vi "Log BoP.vi"(9 "Stop Chat":bool, 10 "Send":bool, 11 "Enter Text":string) -> (3 "Chat Window":string)   [LabVIEW 2017]
uses:
  <vilib>/OPCUA/controls/Write Status.ctl
  <vilib>/OPCUA/controls/NodeId.ctl
  <vilib>/OPCUA/client/Multiple Write String.vi
  <vilib>/OPCUA/NI OPC UA Client.lvlib
panel:
  out "Log Loop":i32
  out "Send Loop":i32
  in  "Node Status":T1 items=["Good"=0, "Uncertain_InitialValue"=1083310080, "Uncertain_LastUsableValue"=1083179008, "Uncertain_SensorNotAccurate"=1083375616, "Uncertain_EngineeringUnitsExceeded"=1083441152, "Bad_NoCommunication"=2150694912, "Bad_NotReadable"=2151284736, "Bad_NotWritable"=2151350272, "Bad_OutOfRange"=2151415808, "Bad_WaitingForInitialData"=2150760448]
  in  "Time Stamp":timestamp
  in  "Node Status":T1 items=["Good"=0, "Uncertain_InitialValue"=1083310080, "Uncertain_LastUsableValue"=1083179008, "Uncertain_SensorNotAccurate"=1083375616, "Uncertain_EngineeringUnitsExceeded"=1083441152, "Bad_NoCommunication"=2150694912, "Bad_NotReadable"=2151284736, "Bad_NotWritable"=2151350272, "Bad_OutOfRange"=2151415808, "Bad_WaitingForInitialData"=2150760448]
  in  "Time Stamp":timestamp
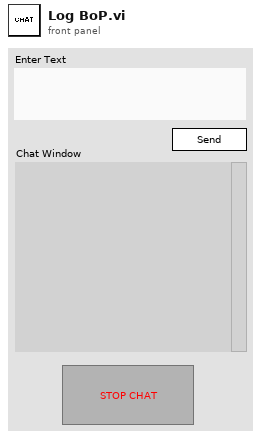
[diagram p1: front panel]
types:
  T1 = typedef "Write Status.ctl" = u32
  T2 = enum16{"open", "replace", "create", "open or create", "replace or create", "replace or create with confirmation"}
  T3 = typedef "OPC UA Client Refnum.ctl" = refnum<k21>
  T4 = typedef "NodeId.ctl" = string
  T5 = cluster{"node ID":T4, "value":string, "timestamp (current time)":timestamp, "node status":T1}
  T6 = cluster{"node ID":T4, "value":string, "timestamp (current time)":timestamp, "node status":T1}[]
  T7 = typedef "Subscription ID.ctl" = u32
  T8 = typedef "Subscription Data Change.ctl" = cluster{"node ID":T4, " value":variant, "timestamp":timestamp, "data type":T9, "status code":T10}
  T9 = typedef "Data Type.ctl" = u16
  T10 = typedef "OPC UA StatusCode.ctl" = u32
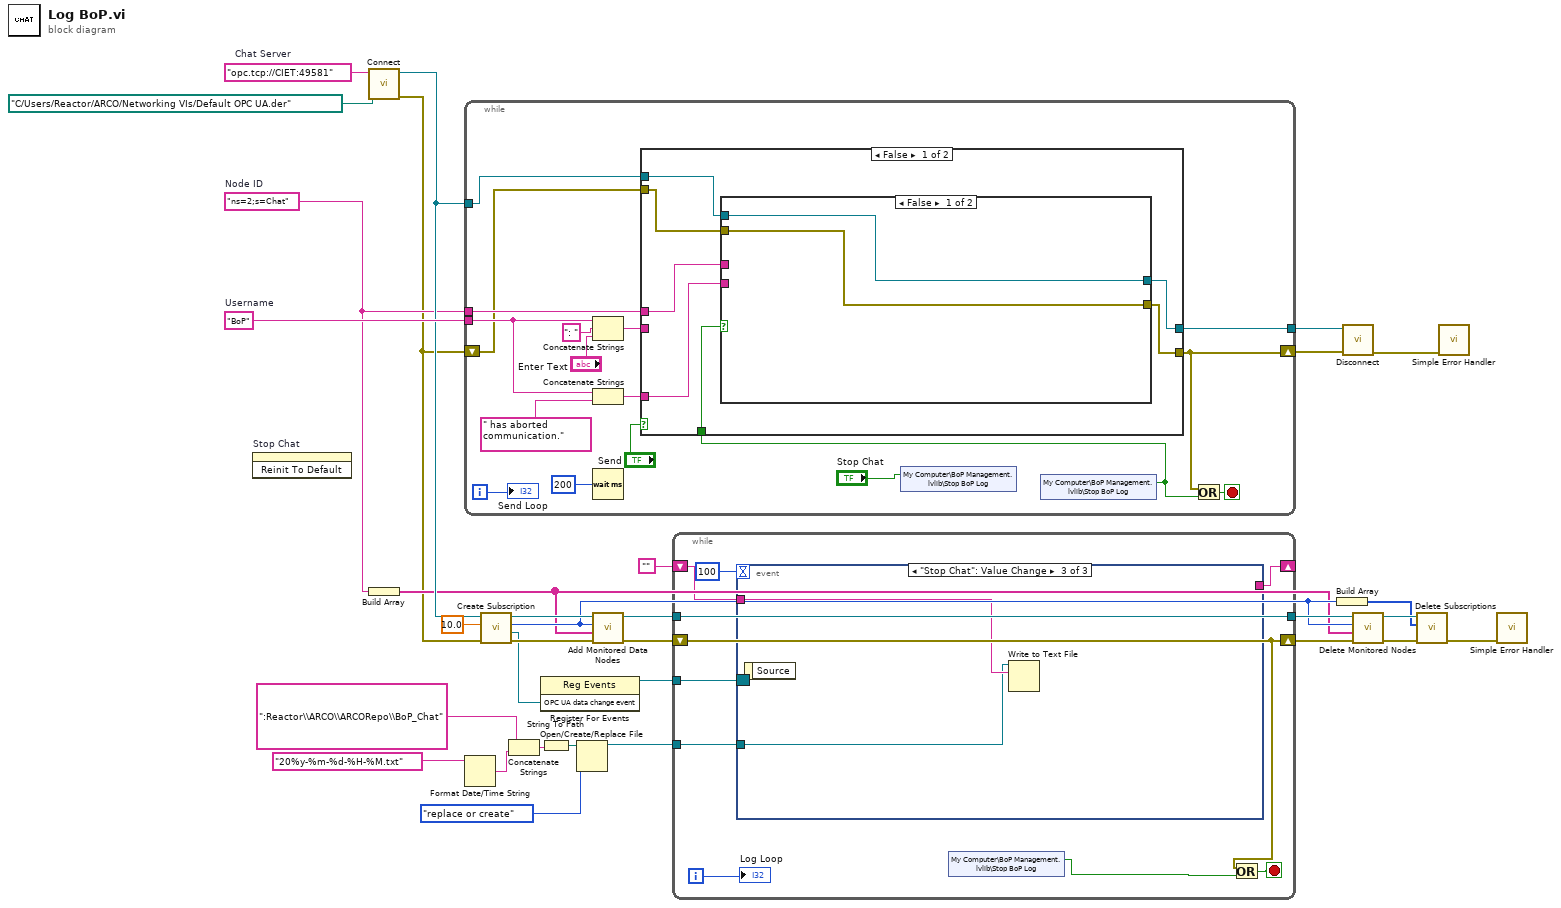
[diagram p0: block diagram]
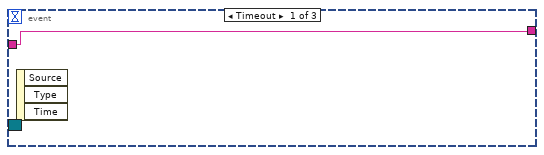
[diagram p2: hidden frame]
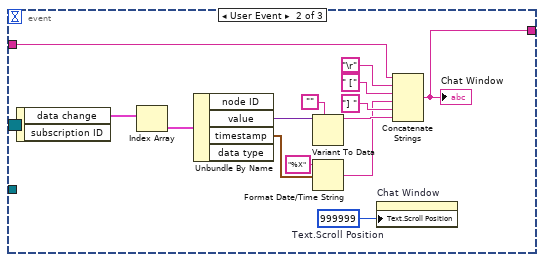
[diagram p3: hidden frame]
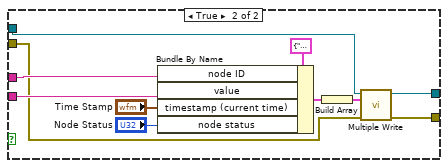
[diagram p4: hidden frame]
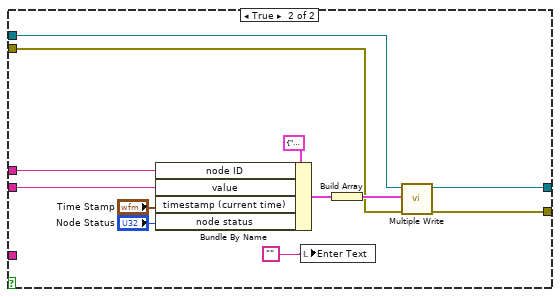
[diagram p5: hidden frame]
diagram:
  w14 = "ns=2;s=Chat"  # Node ID
  w30 = "BoP"  # Username
  w31 = "opc.tcp://CIET:49581"  # Chat Server
  n1 = invoke on="Stop Chat" class="Bool (strict)" method="Reinit To Default"() -> ()  [unwired: 3 in, 3 out]
  n2 = call <vilib>:"Connect.vi"("client certificate file"=path "C:/Users/Reactor/ARCO/Networking VIs/Default OPC UA.der", "server endpoint URL"=w31) -> ("error out"=w4:errorcluster, "OPC UA client refnum out"=w29:T3)  [unwired: 7 in, 1 out]
  n3 = Build Array(w14) -> (w13:string[])
  n4 = while {
    tunnel: w14 -> [w41]
    tunnel: w30 -> [w46]
    tunnel: w29 -> [w39]
    tunnel: [w40] -> w11
    shift-right: [w35] -> w3
    shift-left: w4 -> [w38]
    i -> [w44]
    stop <- w36 stop-if-true
    n5 = Concatenate Strings(w46, ": ", "Enter Text") -> (w42:string)
    n6 = Concatenate Strings(w46, " has aborted communication.") -> (w37:string)
    n7 = Wait (ms)(milliseconds to wait=u32 200) -> ()  [unwired: 1 out]
    n8 = shared-variable "My Computer\\BoP Management.lvlib\\Stop BoP Log"("Stop Chat") -> ()  [unwired: 1 in, 1 out]
    n9 = shared-variable "My Computer\\BoP Management.lvlib\\Stop BoP Log"() -> (w33:bool)  [unwired: 1 in, 1 out]
    n10 = case shown="False" "Send" {
      tunnel: w42 -> [_ w76]
      tunnel: w41 -> [w54 w75]
      tunnel: [w50 w73] -> w40
      tunnel: [w51 w72] -> w35
      tunnel: w39 -> [w52 w71]
      tunnel: w38 -> [w53 w70]
      tunnel: w33 -> [w56 _]
      tunnel: w37 -> [w55 _]
      frame False {
        n11 = case shown="False" w56 {
          tunnel: w55 -> [_ w64]
          tunnel: w54 -> [_ w63]
          tunnel: w53 -> [w57 w62]
          tunnel: w52 -> [w58 w61]
          tunnel: [w58 w60] -> w50
          tunnel: [w57 w59] -> w51
          frame False {
          }
          frame True {
            n12 = Bundle By Name(cluster=T5 {"node ID"="", "value"="", "timestamp (current time)"=timestamp(0 s since 1904-01-01), "node status"=0} ("request"), "node ID"=w63, "value"=w64, "timestamp (current time)"="Time Stamp", "node status"="Node Status") -> (w67:T5)
            n13 = Build Array(w67) -> (w66:T6)
            n14 = call-poly <vilib>:"Multiple Write.vi"("error in (no error)"=w62, "requests"=w66, "OPC UA client refnum in"=w61) -> ("error out"=w59:errorcluster, "OPC UA client refnum out"=w60:T3)  [unwired: 5 in, 2 out]
          }
        }
      }
      frame True {
        n15 = Bundle By Name(cluster=T5 {"node ID"="", "value"="", "timestamp (current time)"=timestamp(0 s since 1904-01-01), "node status"=0} ("request"), "node ID"=w75, "value"=w76, "timestamp (current time)"="Time Stamp", "node status"="Node Status") -> (w79:T5)
        n16 = local write "Enter Text"("") -> ()
        n17 = Build Array(w79) -> (w78:T6)
        n18 = call-poly <vilib>:"Multiple Write.vi"("error in (no error)"=w70, "requests"=w78, "OPC UA client refnum in"=w71) -> ("error out"=w72:errorcluster, "OPC UA client refnum out"=w73:T3)  [unwired: 5 in, 2 out]
      }
    }
    n19 = Or(x=w35, y=w33) -> (x .or. y?=w36:bool)
    "Send Loop" <- w44
  }
  n20 = Format Date/Time String(time format string (%c)="20%y-%m-%d-%H-%M.txt") -> (date/time string=w8:string)  [unwired: 2 in]
  n21 = call <vilib>:"Create Subscription.vi"("error in (no error)"=w4, "publishing interval (1000 ms)"=10.0, "OPC UA client refnum in"=w29) -> ("error out"=w27:errorcluster, "OPC UA data change event"=w26:refnum<user-event>, "subscription ID out"=w18:T7, "OPC UA client refnum out"=w28:T3)  [unwired: 4 in, 1 out]
  n22 = Concatenate Strings(":Reactor\\ARCO\\ARCORepo\\BoP_Chat", w8) -> (w6:string)
  n23 = register-events(w26) -> (reference out=w25:refnum<event-registration>)  [unwired: 2 in, 1 out]
  n24 = String To Path(string=w6) -> (path=w5:path)
  n25 = Open/Create/Replace File(file path (use dialog)=w5, operation (0:open)=T2."replace or create") -> (refnum out=w15:refnum<file>)  [unwired: 4 in, 2 out]
  n26 = call <vilib>:"Add Monitored Data Nodes.vi"("error in (no error)"=w27, "node IDs"=w13, "subscription ID in"=w18, "OPC UA client refnum in"=w28) -> ("error out"=w21:errorcluster, "OPC UA client refnum out"=w23:T3)  [unwired: 4 in, 2 out]
  n27 = while {
    tunnel: w25 -> [w91]
    shift-right: [w89] -> _
    shift-left: "" -> [w90]
    tunnel: w23 -> [w88]
    tunnel: [w88] -> w22
    tunnel: w15 -> [w87]
    shift-right: [w83] -> w2
    shift-left: w21 -> [w83]
    i -> [w86]
    stop <- w84 stop-if-true
    n28 = event shown="[2] \"Stop Chat\": Value Change" {
      selector: w91 -> [_ _ _]
      dyn-events: _ -> [_ _ _]
      timeout: 100 -> [_ _ _]
      tunnel: w90 -> [w92 w95 w108]
      tunnel: [w92 w94 _] -> w89
      tunnel: w87 -> [_ _ w107]
      event Timeout {
        n29 = event-data() -> ()  [unwired: 1 in, 3 out]
      }
      event User Event {
        w93 = u32 999999  # Text.Scroll Position
        n30 = event-data() -> ("data change"=w106:T8[])  [unwired: 1 in, 1 out]
        n31 = Index Array(array=w106) -> (element=w105:T8)  [unwired: 1 in]
        n32 = Unbundle By Name(w105) -> ("value"=w104:variant, "timestamp"=w102:timestamp)  [unwired: 2 out]
        n33 = Variant To Data(type="", Variant=w104) -> (data=w100:string)  [unwired: 1 in, 1 out]
        n34 = Format Date/Time String(time format string (%c)="%X", seconds (now)=w102) -> (date/time string=w98:string)  [unwired: 1 in]
        n35 = property on="Chat Window" class="Str"("Text.Scroll Position"=w93) -> ()  [unwired: 2 in, 2 out]
        n36 = Concatenate Strings(w95, "\r", " [", w98, "] ", w100) -> (w94:string)
        "Chat Window" <- w94
      }
      event "Stop Chat": Value Change {
        n37 = event-data() -> ()  [unwired: 1 in, 1 out]
        n38 = Write to Text File(file (use dialog)=w107, text=w108) -> ()  [unwired: 2 in, 3 out]
      }
    }
    n39 = shared-variable "My Computer\\BoP Management.lvlib\\Stop BoP Log"() -> (w82:bool)  [unwired: 1 in, 1 out]
    n40 = Or(x=w83, y=w82) -> (x .or. y?=w84:bool)
    "Log Loop" <- w86
  }
  n41 = Build Array(w18) -> (w17:T7[])
  n42 = call <vilib>:"Disconnect.vi"("error in (no error)"=w3, "OPC UA client refnum in"=w11) -> ("error out"=w32:errorcluster)  [unwired: 9 in]
  n43 = call <vilib>:"Delete Monitored Nodes.vi"("error in (no error)"=w2, "node IDs"=w13, "subscription ID in"=w18, "OPC UA client refnum in"=w22) -> ("error out"=w19:errorcluster, "OPC UA client refnum out"=w20:T3)  [unwired: 3 in, 3 out]
  n44 = call <vilib>:"Delete Subscriptions.vi"("error in (no error)"=w19, "subscription IDs"=w17, "OPC UA client refnum in"=w20) -> ("error out"=w16:errorcluster)  [unwired: 6 in, 2 out]
  n45 = call <vilib>:"Simple Error Handler.vi"("error in (no error)"=w32) -> ()  [unwired: 4 in, 5 out]
  n46 = call <vilib>:"Simple Error Handler.vi"("error in (no error)"=w16) -> ()  [unwired: 4 in, 5 out]
